vi "register_as_observer.vi"(8 "error in (no error)":errorcluster, 11 "GenericToplevelComponent in":refnum<class "GenericToplevelComponent.lvclass">) -> (0 "error out":errorcluster, 3 "GenericToplevelComponent out":refnum<class "GenericToplevelComponent.lvclass">)   [LabVIEW 2010, in "GenericToplevelComponent.lvclass"]
uses:
  GenericToplevelComponent.lvclass
  GenericToplevelComponent.lvclass/GenericToplevelComponent.ctl
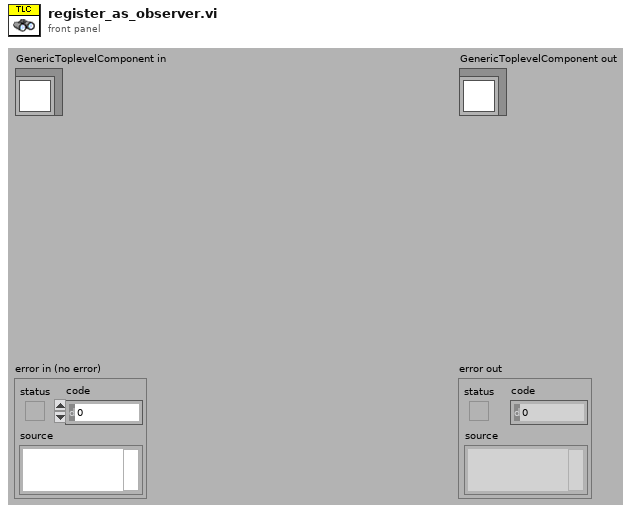
[diagram p1: front panel]
types:
  T1 = typedef "top-level_component_type_enum.ctl" = enum16{"undefined", "ImagingMode", "ScanHead", "DAQ", "ImageAssembler", "Display", "DataCollection", "Analyser", "Stimulator", "ExperimentController", "Instrument", "Stage"}
  T2 = typedef "GenericToplevelComponent.lvclass/common_trigger_enum.ctl" = enum16{"NULL", "initialise", "terminate", "fetch command", "fetch data", "attach observer", "register as observer", "detach observer", "acknowledge", "start", "stop", "sweep started", "sweep finished", "experiment started", "experiment stopped"}
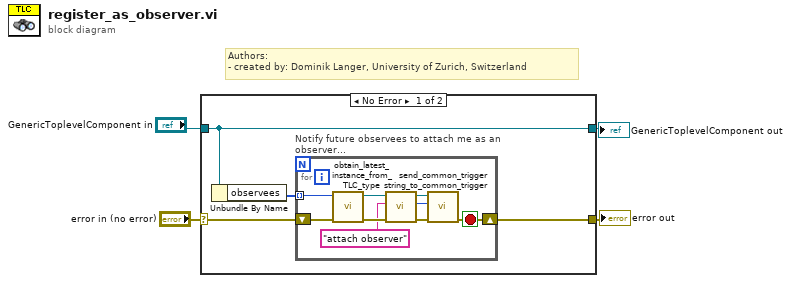
[diagram p0: block diagram]
diagram:
  # "Authors: \n- created by: Dominik Langer, University of Zurich, Switzerland"
  n1 = case shown="No Error" "error in (no error)" {
    selector: "error in (no error)" -> [w7 w19]
    tunnel: [w6 w19] -> w3
    tunnel: [w8 w18] -> w4
    tunnel: "GenericToplevelComponent in" -> [w8 w18]
    frame No Error {
      n2 = Unbundle By Name(w8) -> ("observees"=w5:T1[])
      n3 = for "Notify future observees to attach me as an observer..." {
        tunnel: w5 -> [w16] mode=indexing
        shift-right: [w15] -> w6
        shift-left: w7 -> [w17]
        stop <- w15 stop-if-true
        n4 = call "obtain_latest_instance_from_TLC_type.vi"("error in (no error)"=w17, "top-level component type"=w16) -> ("error out"=w14:errorcluster, "GenericToplevelComponent.lvclass"=w12:refnum<class "GenericToplevelComponent.lvclass">)  [unwired: 8 in]
        n5 = call-dynamic "string_to_common_trigger.vi"("error in (no error)"=w14, "trigger string"="attach observer", "GenericToplevelComponent in"=w12) -> ("error out"=w13:errorcluster, "trigger"=w10:T2, "GenericToplevelComponent out"=w11:refnum<class "GenericToplevelComponent.lvclass">)  [unwired: 6 in]
        n6 = call-dynamic "send_common_trigger.vi"("error in (no error)"=w13, "trigger"=w10, "GenericToplevelComponent in"=w11) -> ("error out"=w15:errorcluster)  [unwired: 6 in, 2 out]
      }
    }
    frame Error {
    }
  }
  "error out" <- w3
  "GenericToplevelComponent out" <- w4
